vi "Read Queue Ref.vi"(8 "error in":errorcluster, 11 "QueueMessageTransport in":refnum<class "QueueMessageTransport.lvclass">) -> (0 "error out":errorcluster, 2 "Queue Ref":refnum<queue>, 3 "QueueMessageTransport out":refnum<class "QueueMessageTransport.lvclass">)   [LabVIEW 2016, in "QueueMessageTransport.lvclass"]
doc: "QueueMessageTransport <B>Private</B> method for accessing class private data.\n\n**Author: Stas Legedza"
uses:
  QueueMessageTransport.lvclass
  IMessagePayload/IMessagePayload.lvclass
  QueueMessageTransport.lvclass/QueueMessageTransport.ctl
panel:
  # "INPUTS"
  # "OUTPUTS"
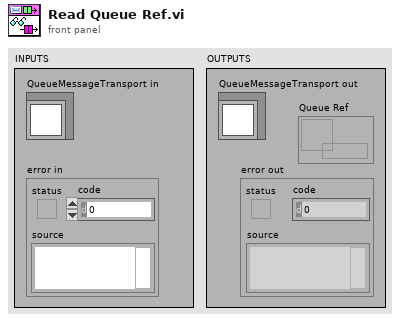
[diagram p1: front panel]
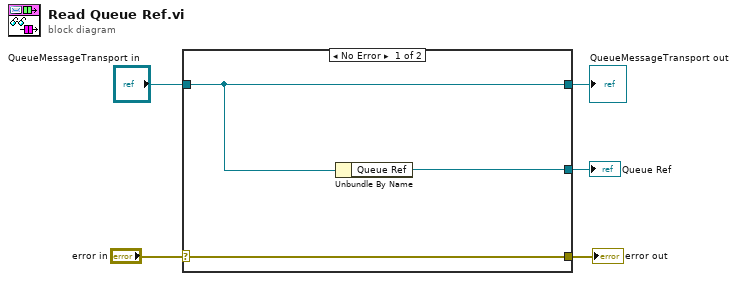
[diagram p0: block diagram]
diagram:
  n1 = case shown="No Error" "error in" {
    selector: "error in" -> [w8 w9]
    tunnel: [w8 w9] -> w4
    tunnel: [w7 w10] -> w2
    tunnel: "QueueMessageTransport in" -> [w7 w10]
    tunnel: [w6 _] -> w1
    frame No Error {
      n2 = Unbundle By Name(w7) -> ("Queue Ref"=w6:refnum<queue>)
    }
    frame Error {
    }
  }
  "error out" <- w4
  "QueueMessageTransport out" <- w2
  "Queue Ref" <- w1
